vi "Test Analog Input.vi"() -> ()   [LabVIEW 2013]
uses:
  <vilib>/DAQmx/create/channels.llb/DAQmx Create Channel (AI-Voltage-Basic).vi
  <vilib>/DAQmx/configure/timing.llb/DAQmx Timing (Sample Clock).vi
  <vilib>/DAQmx/read.llb/DAQmx Read (Analog 1D Wfm NChan NSamp).vi
panel:
  out "x-y":dbl
  out "Waveform Chart":dbl(graph)
  out "Waveform Graph":waveform(dbl)[](graph)
  in  "maximum value":dbl=5.0 format="%0.2f"
  in  "minimum value":dbl=-5.0 format="%0.2f"
  out "Numeric":i32
  in  "rate":dbl=1000.0 format="%0.2f"
  in  "stop":bool
  in  "number of samples per channel":i32=-1
  in  "physical channels":tag
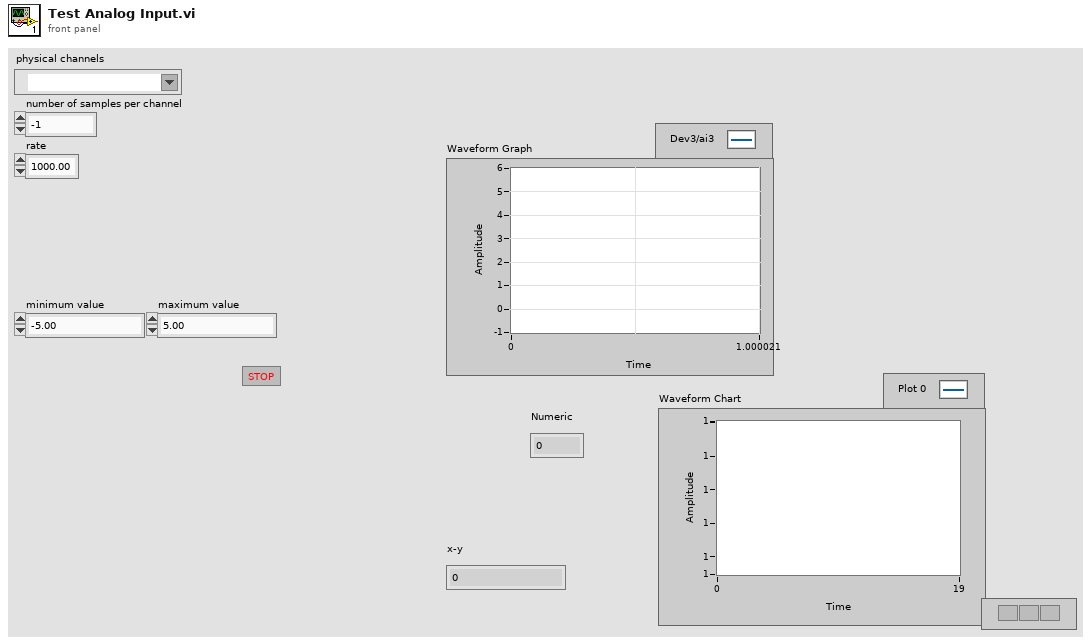
[diagram p1: front panel]
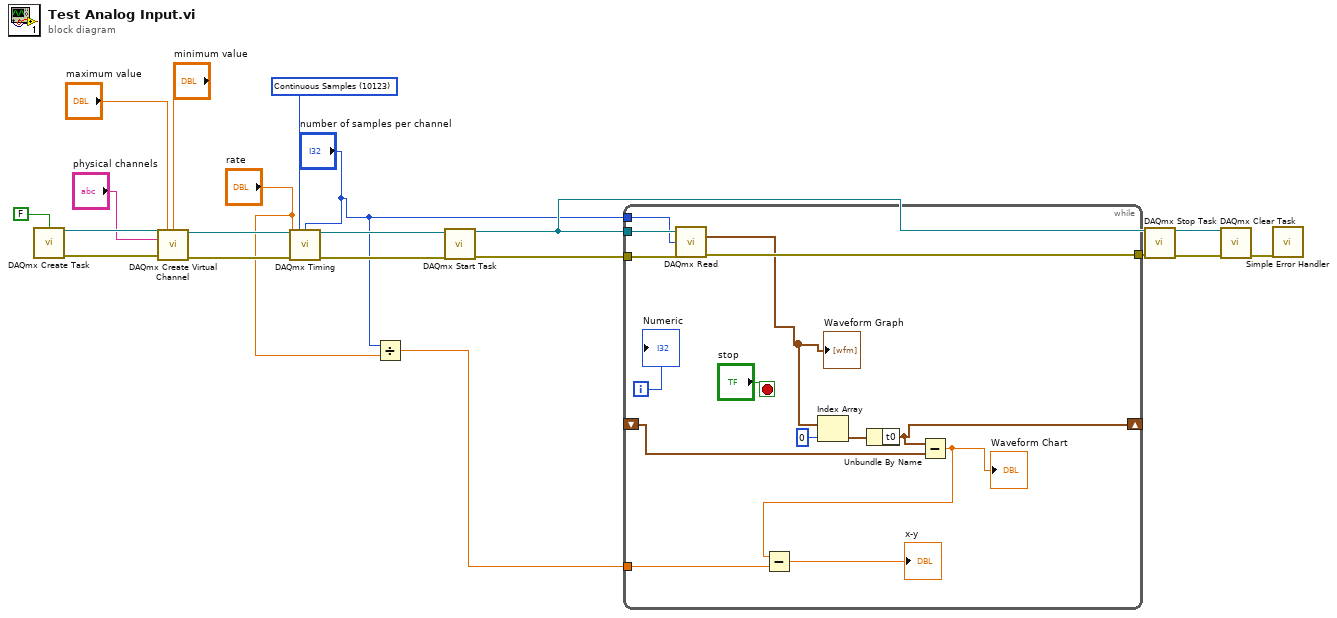
[diagram p0: block diagram]
diagram:
  w4 = 10123 items=["Finite Samples"=10178, "Continuous Samples"=10123, "Hardware Timed Single Point"=12522] ("sample mode")
  n1 = call <vilib>:"DAQmx Create Task.vi"("auto cleanup"=FALSE) -> ("task out"=w19:refnum<k21>, "error out"=w17:errorcluster)  [unwired: 13 in]
  n2 = call-poly <vilib>:"DAQmx Create Virtual Channel.vi"("task in"=w19, "maximum value"="maximum value", "minimum value"="minimum value", "physical channels"="physical channels", "error in"=w17) -> ("task out"=w16:refnum<k21>, "error out"=w15:errorcluster)  [unwired: 9 in]
  n3 = call-poly <vilib>:"DAQmx Timing.vi"("task/channels in"=w16, "sample mode"=w4, "samples per channel"="number of samples per channel", "rate"="rate", "error in"=w15) -> ("task out"=w14:refnum<k21>, "error out"=w13:errorcluster)  [unwired: 9 in]
  n4 = Divide(x="number of samples per channel", y="rate") -> (x/y=w1:dbl)
  n5 = call <vilib>:"DAQmx Start Task.vi"("task/channels in"=w14, "error in"=w13) -> ("task out"=w5:refnum<k21>, "error out"=w12:errorcluster)  [unwired: 12 in]
  n6 = while {
    tunnel: w5 -> [w34]
    tunnel: w12 -> [w33]
    tunnel: [w32] -> w10
    tunnel: "number of samples per channel" -> [w29]
    shift-right: [w25] -> _
    shift-left: _ -> [w24]
    tunnel: w1 -> [w23]
    i -> [w30]
    stop <- "stop" stop-if-true
    n7 = call-poly <vilib>:"DAQmx Read.vi"("task/channels in"=w34, "number of samples per channel"=w29, "error in"=w33) -> ("data"=w28:waveform(dbl)[], "error out"=w32:errorcluster)  [unwired: 10 in, 1 out]
    "Waveform Graph" <- w28
    n8 = Index Array(array=w28, index=0) -> (element=w26:waveform(dbl))
    n9 = Unbundle By Name(w26) -> ("t0"=w25:timestamp)
    n10 = Subtract(x=w25, y=w24) -> (x-y=w22:dbl)
    "Waveform Chart" <- w22
    n11 = Subtract(x=w22, y=w23) -> (x-y=→"x-y":dbl)
    "Numeric" <- w30
  }
  n12 = call <vilib>:"DAQmx Stop Task.vi"("task/channels in"=w5, "error in"=w10) -> ("task out"=w11:refnum<k21>, "error out"=w9:errorcluster)  [unwired: 12 in]
  n13 = call <vilib>:"DAQmx Clear Task.vi"("task in"=w11, "error in"=w9) -> ("error out"=w8:errorcluster)  [unwired: 13 in]
  n14 = call <vilib>:"Simple Error Handler.vi"("error in (no error)"=w8) -> ()  [unwired: 4 in, 5 out]
